vi "Add File to Target.vi"(8 "error in (no error)":errorcluster, 9 "Flie Path":path, 10 "Target Name":string, 11 "Project Sync Tools in":refnum<class "Project Sync Tools.lvclass">) -> (0 "error out":errorcluster, 3 "Project Sync Tools out":refnum<class "Project Sync Tools.lvclass">)   [LabVIEW 2019, in "Project Sync Tools.lvclass"]
uses:
  Project Sync Tools.lvclass
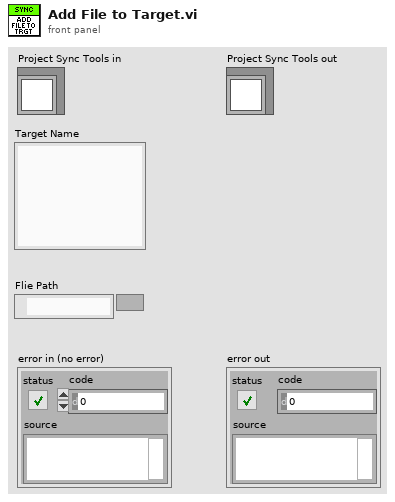
[diagram p1: front panel]
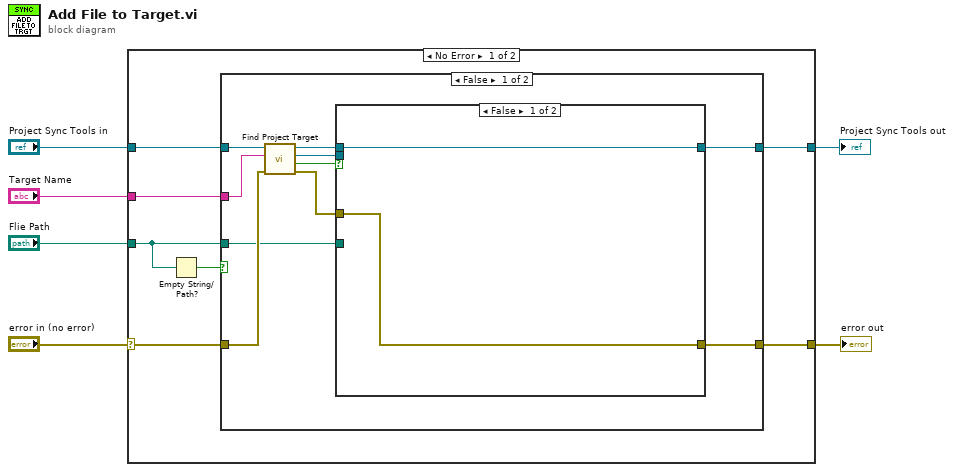
[diagram p0: block diagram]
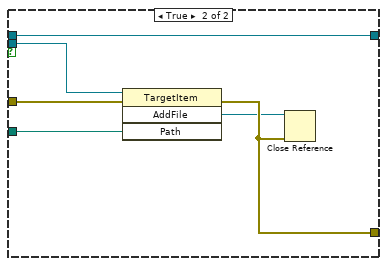
[diagram p2: hidden frame]
diagram:
  n1 = case shown="No Error" "error in (no error)" {
    selector: "error in (no error)" -> [w9 w34]
    tunnel: [w13 w34] -> w6
    tunnel: "Project Sync Tools in" -> [w12 w35]
    tunnel: "Flie Path" -> [w8 _]
    tunnel: [w10 w35] -> w3
    tunnel: "Target Name" -> [w11 _]
    frame No Error {
      n2 = Empty String/Path?(string/path=w8) -> (empty?=w7:bool)
      n3 = case shown="False" w7 {
        tunnel: [w23 w32] -> w13
        tunnel: w12 -> [w22 w33]
        tunnel: w11 -> [w21 _]
        tunnel: [w16 w33] -> w10
        tunnel: w9 -> [w15 w32]
        tunnel: w8 -> [w14 _]
        frame False {
          n4 = call "Find Project Target.vi"("error in (no error)"=w15, "Target Name"=w21, "Project Sync Tools in"=w22) -> ("error out"=w20:errorcluster, "Found ?"=w19:bool, "TargetItem out"=w18:refnum<vi>, "Project Sync Tools out"=w17:refnum<class "Project Sync Tools.lvclass">)  [unwired: 5 in]
          n5 = case shown="False" w19 {
            tunnel: [w24 w31] -> w23
            tunnel: w14 -> [_ w29]
            tunnel: w20 -> [w24 w28]
            tunnel: w18 -> [_ w27]
            tunnel: w17 -> [w25 w26]
            tunnel: [w25 w26] -> w16
            frame False {
            }
            frame True {
              n6 = invoke class="TargetItem" method="AddFile"(reference=w27, error in=w28, "Path"=w29) -> (error out=w31:errorcluster, "AddFile"=w30:refnum<vi>)  [unwired: 1 in, 2 out]
              n7 = Close Reference(reference=w30, error in (no error)=w31) -> ()  [unwired: 1 out]
            }
          }
        }
        frame True {
        }
      }
    }
    frame Error {
    }
  }
  "error out" <- w6
  "Project Sync Tools out" <- w3
